vi "fitCoefficient.vi"(10 "n":dbl, 11 "a":dbl) -> (2 "d":dbl, 3 "c":dbl)   [LabVIEW 2016]
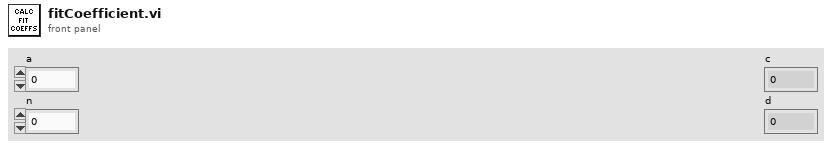
[diagram p1: front panel]
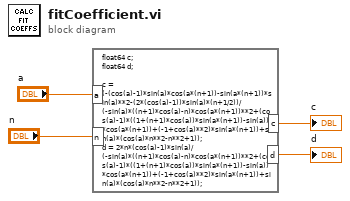
[diagram p0: block diagram]
diagram:
  n1 = formula code="float64 c;\nfloat64 d;\n\nc =  (-(cos(a)-1)*sin(a)*cos(a*(n+1))-sin(a*(n+1))*sin(a)**2-(2*(cos(a)-1))*sin(a)*(n+1/2))/(-sin(a)*((n+1)*cos(a)-n)*cos(a*(n+1))**2+(cos(a)-1)*((1+(n+1)*cos(a))*sin(a*(n+1))-sin(a))*cos(a*(n+1))+(-1+cos(a)**2)*sin(a*(n+1))+sin(a)*(cos(a)*n**2-n**2+1));\nd = 2*n*(cos(a)-1)*sin(a)/(-sin(a)*((n+1)*cos(a)-n)*cos(a*(n+1))**2+(cos(a)-1)*((1+(n+1)*cos(a))*sin(a*(n+1))-sin(a))*cos(a*(n+1))+(-1+cos(a)**2)*sin(a*(n+1))+sin(a)*(cos(a)*n**2-n**2+1));"("a"="a", "n"="n") -> ("c"=→"c":dbl, "d"=→"d":dbl)
